vi "StringToIni.vi"(8 "ErrorArray in":errorcluster[](array[cluster]), 10 "StringRefArray":refnum<vi>[](array[refnum]), 11 "IniFileRef in":T1) -> (0 "ErrorArray out":errorcluster[](array[cluster]), 3 "InifileRef out":T1)   [LabVIEW 2014, in "Ini_lib.lvlib"]
uses:
  Ini_lib.lvlib
  <vilib>/Utility/config.llb/Config Data RefNum.ctl
  <userlib>/NIST/NISTErrorLib/NISTErrorLib.lvlib
  <vilib>/Utility/config.llb/NI_LVConfig.lvlib
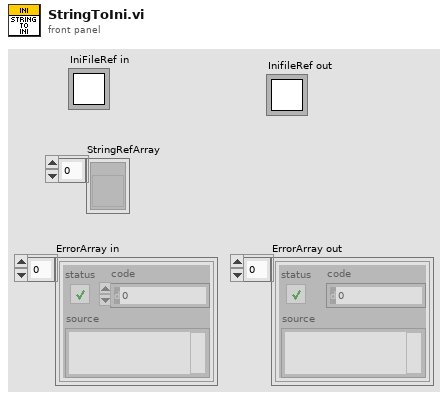
[diagram p1: front panel]
types:
  T1 = typedef "NI_LVConfig.lvlib/Config Data RefNum.ctl" = refnum<k1>
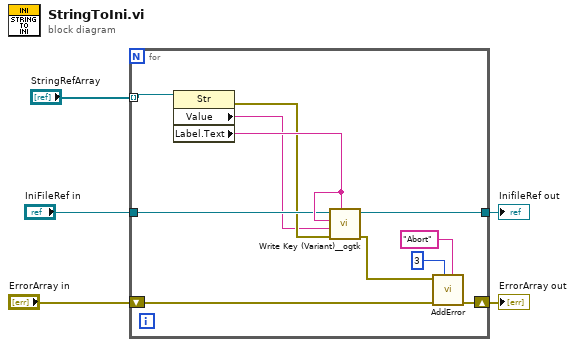
[diagram p0: block diagram]
diagram:
  n1 = for {
    tunnel: "StringRefArray" -> [w16] mode=indexing
    tunnel: "IniFileRef in" -> [w14]
    shift-right: [w10] -> w2
    shift-left: "ErrorArray in" -> [w11]
    tunnel: [w9] -> w4
    n2 = property class="Str"(reference=w16) -> (error out=w7:errorcluster, "Value"=w6:string, "Label.Text"=w15:string)  [unwired: 1 in, 1 out]
    n3 = call <userlib>:"Write Key (Variant)__ogtk.vi"("section"=w15, "error in (no error)"=w7, "key-value"=w6, "key (optional)"=w15, "refnum"=w14) -> ("error out"=w8:errorcluster, "refnum out"=w9:T1)  [unwired: 5 in]
    n4 = call <userlib>:"AddError.vi"("Severity"="Abort", "Priority"=u8 3, "ErrorArray"=w11, "error in (no error)"=w8) -> ("ErrorArray"=w10:errorcluster[])  [unwired: 6 in, 1 out]
  }
  "ErrorArray out" <- w2
  "InifileRef out" <- w4
